vi "Check Sum Test_Initial.vi"(11 "ToolString Input":string="$AGENT,53,VS-62U009+VS-69W014*71") -> (1 "ToolStringOut_Scan":string, 2 "ChkSum":string, 3 "x = y?":bool)   [LabVIEW 2019]
uses:
  LLB/Commonly VI/Main Glb.vi
  LLB/Commonly VI.lvlib
panel:
  out "Array":string[](array[string])
  out "ChkSum2":string
  out "ChkSum1":string
  out "ASCII 格式輸出 2":string
  out "ASCII 格式輸出":string
  out "number 3":u32
  out "number 2":u32
  out "Rad In Reg 2":string
  out "hex integer string":string[](array[string])
  out "unsigned byte array":u8[](array[numeric]) format="%x"
  out "Rad In Reg":string
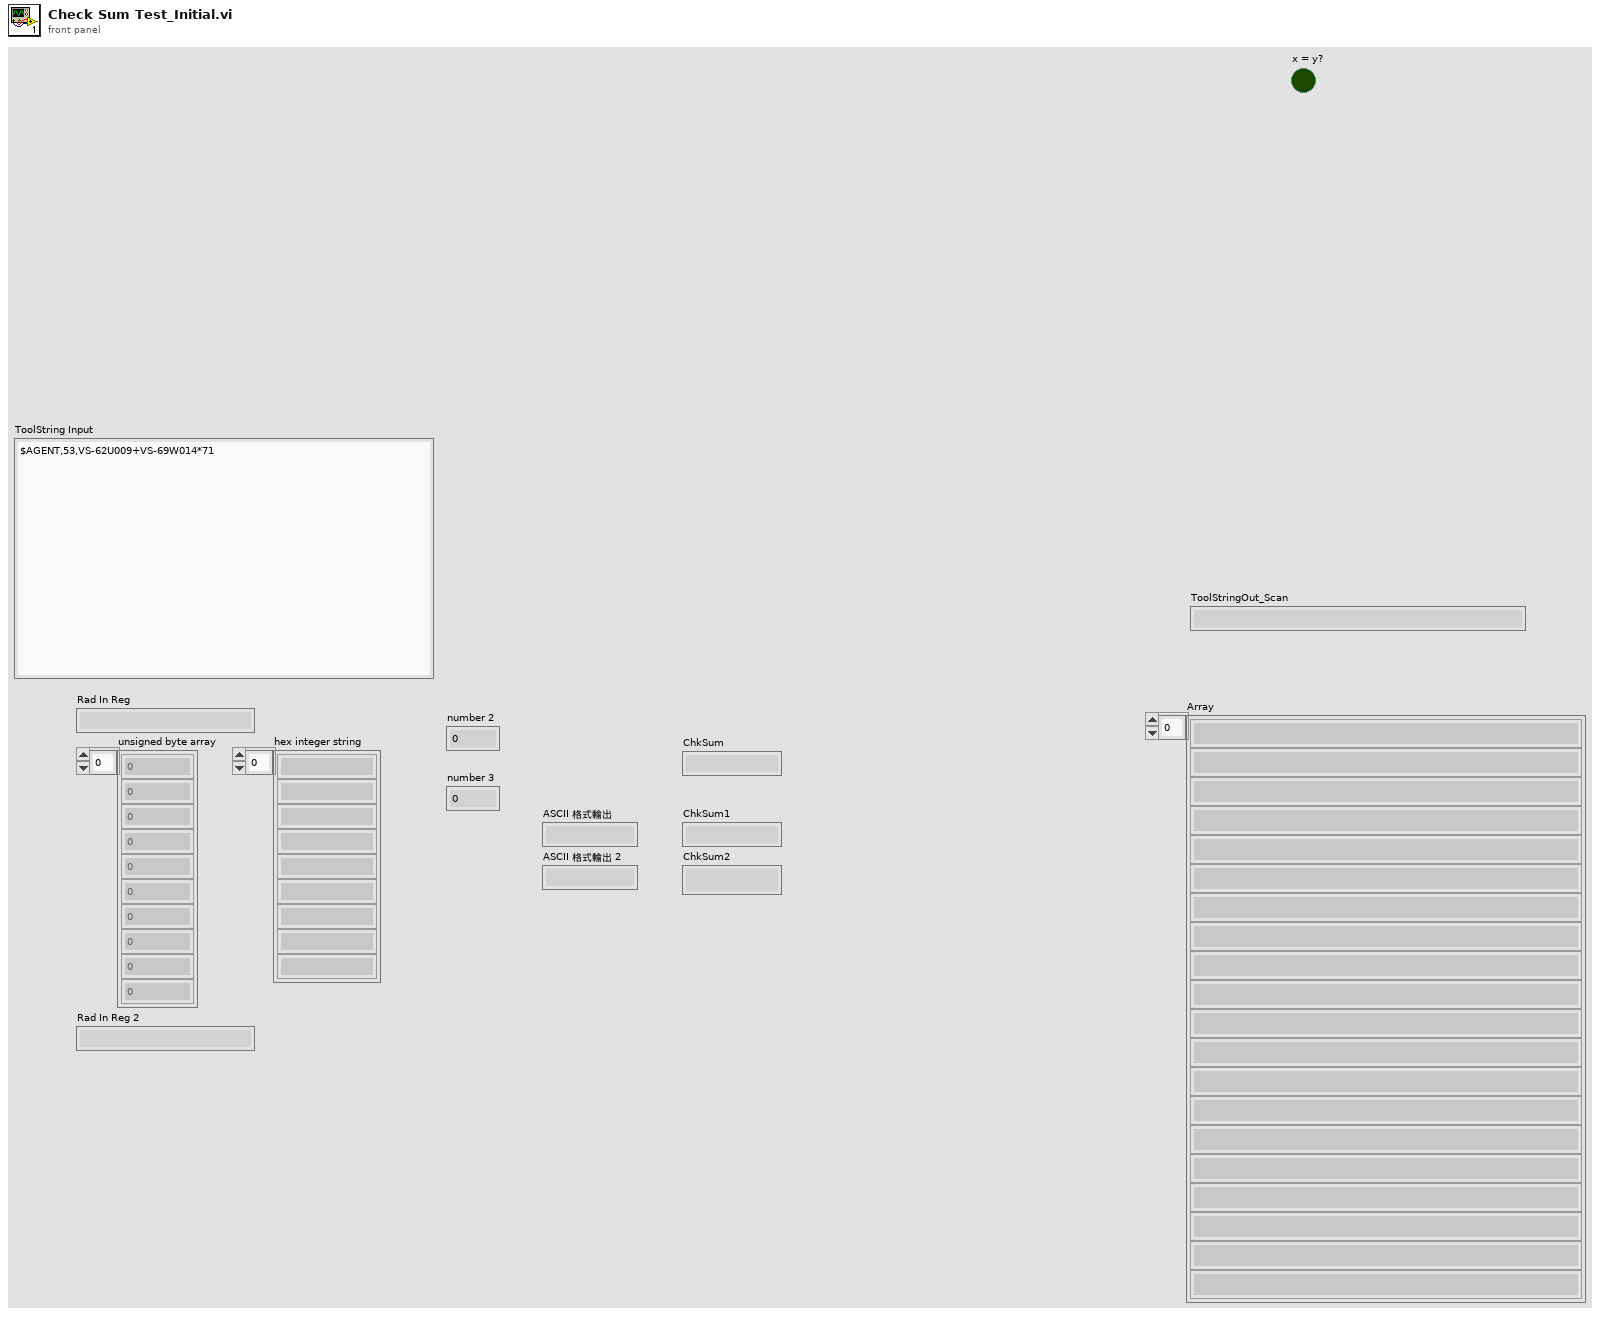
[diagram p1: front panel]
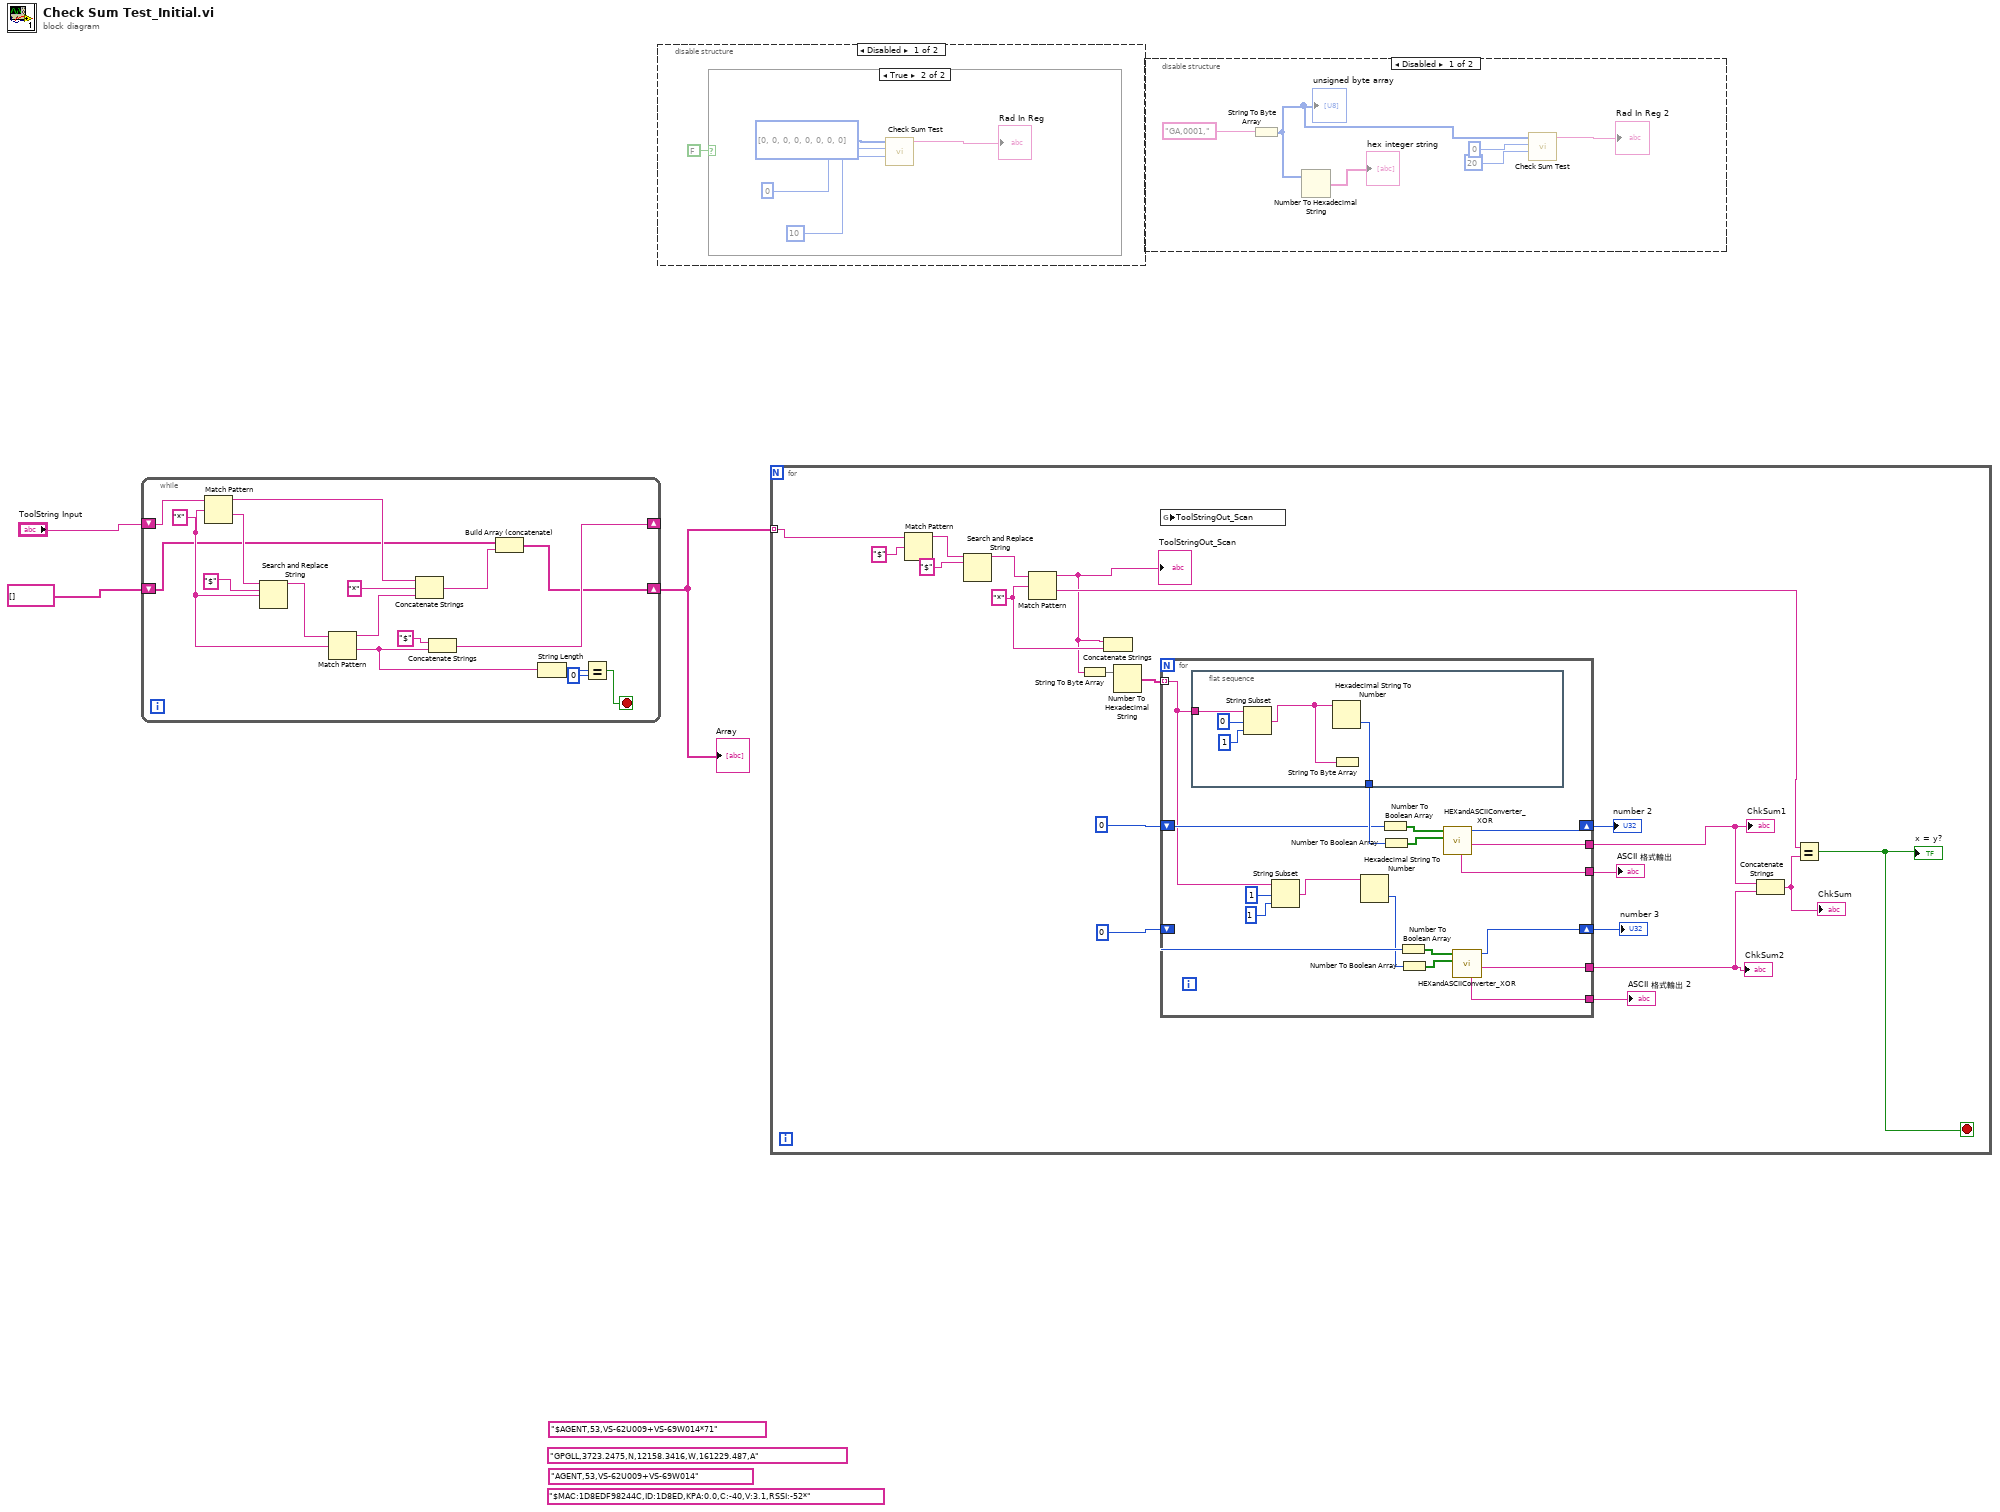
[diagram p0: block diagram]
diagram:
  (unwired) "$AGENT,53,VS-62U009+VS-69W014*71"
  (unwired) "$MAC:1D8EDF98244C,ID:1D8ED,KPA:0.0,C:-40,V:3.1,RSSI:-52*"
  (unwired) "GPGLL,3723.2475,N,12158.3416,W,161229.487,A"
  (unwired) "AGENT,53,VS-62U009+VS-69W014"
  n1 = while {
    shift-right: [w11] -> _
    shift-left: "ToolString Input" -> [w12]
    shift-right: [w8] -> w2
    shift-left: string[] [] -> [w10]
    stop <- w4 stop-if-true
    w18 = "*" ("regular expression")
    n2 = Match Pattern(string=w12, regular expression=w18) -> (before substring=w16:string, after substring=w17:string)  [unwired: 1 in, 2 out]
    n3 = Search and Replace String(input string=w17, search string="$" ("regular expression"), replace string=w18) -> (result string=w19:string)  [unwired: 5 in, 3 out]
    n4 = Match Pattern(string=w19, regular expression=w18) -> (before substring=w14:string, after substring=w5:string)  [unwired: 1 in, 2 out]
    n5 = Concatenate Strings(w16, "*" ("string"), w14) -> (w9:string)
    n6 = Concatenate Strings("$" ("regular expression"), w5) -> (w11:string)
    n7 = Build Array (concatenate)(w10, w9) -> (w8:string[])
    n8 = String Length(string=w5) -> (length=w7:i32)
    n9 = Equal?(x=w7, y=0) -> (x = y?=w4:bool)
  }
  "Array" <- w2
  n10 = disable-structure shown="Disabled" {
    frame Disabled {
      n11 = case shown="True" FALSE {
        frame False {
        }
        frame True {
          n12 = call "Check Sum Test.vi"("length"=10, "index"=0, "Input Registers Arr"=u16[] [0, 0, 0, 0, 0, 0, 0, 0]) -> ("Rad In Reg"=→"Rad In Reg":string)  [unwired: 8 in]
        }
      }
    }
    frame Enabled {
    }
  }
  n13 = for {
    tunnel: w2 -> [w28] mode=indexing
    stop <- w27 stop-if-true
    w33 = "*" ("regular expression")
    n14 = Match Pattern(string=w28, regular expression="$") -> (before substring=w35:string)  [unwired: 1 in, 3 out]
    n15 = Search and Replace String(input string=w35, search string="$" ("regular expression")) -> (result string=w34:string)  [unwired: 6 in, 3 out]
    n16 = Match Pattern(string=w34, regular expression=w33) -> (before substring=w26:string, after substring=w30:string)  [unwired: 1 in, 2 out]
    "ToolStringOut_Scan" <- w26
    n17 = String To Byte Array(string=w26) -> (unsigned byte array=w41:u8[])
    n18 = Concatenate Strings(w26, w33) -> ()  [unwired: 1 out]
    n19 = Number To Hexadecimal String(2:w41) -> (0:w38:string[])  [unwired: 1 in]
    n20 = global read "Main Glb.vi" "ToolStringOut_Scan"() -> ()  [unwired: 1 in]
    n21 = for {
      tunnel: w38 -> [w55] mode=indexing
      shift-right: [w59] -> w44
      shift-left: 0 -> [w60]
      shift-right: [w50] -> w42
      shift-left: 0 -> [w52]
      tunnel: [w49] -> w40
      tunnel: [w48] -> w39
      tunnel: [w47] -> w32
      tunnel: [w46] -> w31
      n22 = flat-sequence {
        tunnel: w55 -> [w66]
        tunnel: [w64] -> w61
        frame #0 {
          n23 = String Subset(string=w66, offset (0)=0, length (rest)=1) -> (substring=w65:string)
          n24 = Hexadecimal String To Number(string=w65) -> (number=w64:u32)  [unwired: 2 in, 1 out]
          n25 = String To Byte Array(string=w65) -> ()  [unwired: 1 out]
        }
      }
      n26 = String Subset(string=w55, offset (0)=1, length (rest)=1) -> (substring=w58:string)
      n27 = Hexadecimal String To Number(string=w58) -> (number=w51:u32)  [unwired: 2 in, 1 out]
      n28 = Number To Boolean Array(number=w60) -> (Boolean array=w63:bool[])
      n29 = Number To Boolean Array(number=w61) -> (Boolean array=w62:bool[])
      n30 = Number To Boolean Array(number=w52) -> (Boolean array=w53:bool[])
      n31 = Number To Boolean Array(number=w51) -> (Boolean array=w54:bool[])
      n32 = call "HEXandASCIIConverter_XOR.vi"("Boolean array2 in"=w62, "Boolean array1 in"=w63) -> ("hex integer string"=w47:string, "number"=w59:u32, "ASCII 格式輸出"=w49:string)  [unwired: 6 in, 1 out]
      n33 = call "HEXandASCIIConverter_XOR.vi"("Boolean array2 in"=w54, "Boolean array1 in"=w53) -> ("hex integer string"=w46:string, "number"=w50:u32, "ASCII 格式輸出"=w48:string)  [unwired: 6 in, 1 out]
    }
    "number 2" <- w44
    "number 3" <- w42
    "ASCII 格式輸出" <- w40
    "ASCII 格式輸出 2" <- w39
    "ChkSum1" <- w32
    "ChkSum2" <- w31
    n34 = Concatenate Strings(w32, w31) -> (w29:string)
    "ChkSum" <- w29
    n35 = Equal?(x=w30, y=w29) -> (x = y?=w27:bool)
    "x = y?" <- w27
  }
  n36 = disable-structure shown="Disabled" {
    frame Disabled {
      n37 = String To Byte Array(string="GA,0001,") -> (unsigned byte array=w72:u8[])
      "unsigned byte array" <- w72
      n38 = Number To Hexadecimal String(2:w72) -> (0:→"hex integer string":string[])  [unwired: 1 in]
      n39 = call "Check Sum Test.vi"("length"=20, "index"=0, "Input Registers Arr"=w72) -> ("Rad In Reg"=→"Rad In Reg 2":string)  [unwired: 8 in]
    }
    frame Enabled {
    }
  }
